vi "GFBuildMagTriggerWaveForm.vi"(3 "error in":errorcluster, 4 "Enable Array":bool[](array[boolean])=[TRUE, TRUE, TRUE, TRUE, TRUE, TRUE, TRUE], 5 "Chan Delays":dbl[](array[numeric])=[-0.8, -0.9, -0.7] format="%.6f", 6 "task in":refnum<k21>="USB-MagAndTrigFire") -> (0 "error out":errorcluster, 1 "Digital Waveform Graph":digitalwaveform[](graph), 2 "task out":refnum<k21>="USB-MagAndTrigFire")   [LabVIEW 2016]
doc: "Magnet timing pulses should be input relative to fast fire pulse, at most 2 s behind (-2 to 0 s)"
uses:
  <vilib>/Waveform/DWDTOps.llb/DWDT Boolean Array to Digital.vi
  <resource>/objmgr/daqmx.rc
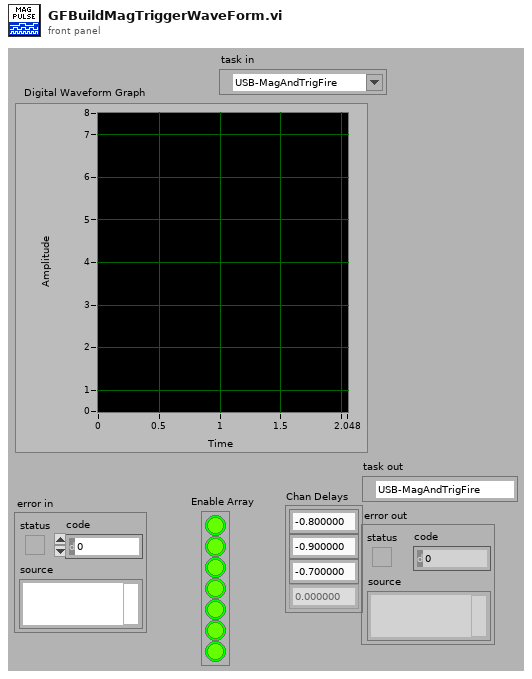
[diagram p1: front panel]
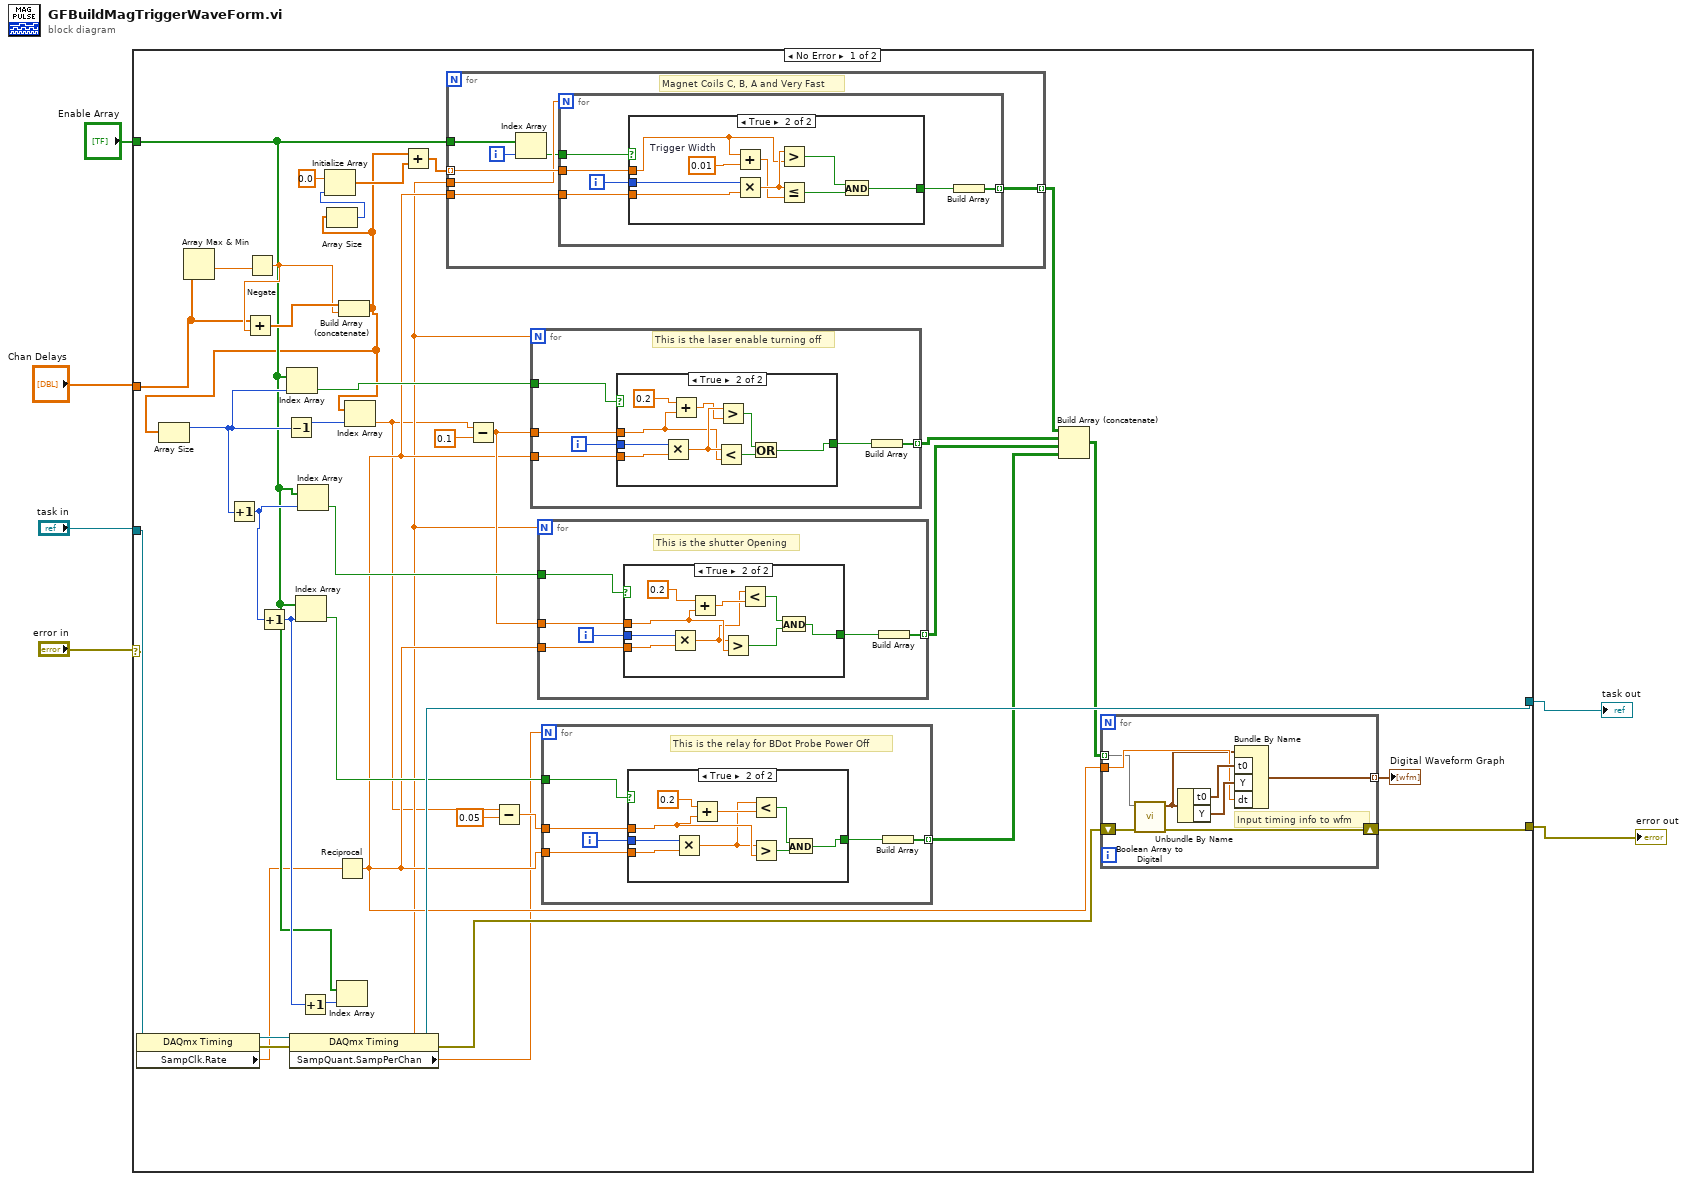
[diagram p0: block diagram]
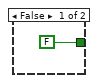
[diagram p2: hidden frame]
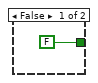
[diagram p3: hidden frame]
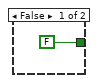
[diagram p4: hidden frame]
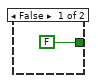
[diagram p5: hidden frame]
diagram:
  n1 = case shown="No Error" "error in" {
    selector: "error in" -> [w42 w125]
    tunnel: "task in" -> [w43 w126]
    tunnel: [w39 w126] -> w5
    tunnel: [w45 w125] -> w3
    tunnel: "Chan Delays" -> [w31 _]
    tunnel: "Enable Array" -> [w14 _]
    frame No Error {
      n2 = property class="DAQmx Timing"(reference=w43, error in=w42) -> (reference out=w41:refnum<k21>, error out=w40:errorcluster, "SampClk.Rate"=w12:dbl)
      n3 = Array Max & Min(array=w31) -> (min value=w34:dbl)  [unwired: 3 out]
      n4 = Negate(x=w34) -> (-x=w32:dbl)
      n5 = Add(x=w31, y=w32) -> (x+y=w33:dbl[])
      n6 = property class="DAQmx Timing"(reference=w41, error in=w40) -> (reference out=w39:refnum<k21>, error out=w25:errorcluster, "SampQuant.SampPerChan"=w17:dbl)
      n7 = Reciprocal(x=w12) -> (1/x=w21:dbl)
      n8 = Build Array (concatenate)(w33, w32) -> (w9:dbl[])
      n9 = Array Size(array=w9) -> (size(s)=w20:i32)
      n10 = Increment(x=w20) -> (x+1=w26:i32)
      n11 = Increment(x=w26) -> (x+1=w15:i32)
      n12 = Decrement(x=w20) -> (x-1=w38:i32)
      n13 = Index Array(array=w14, index=w20) -> (element=w30:bool)
      n14 = Index Array(array=w14, index=w15) -> (element=w24:bool)
      n15 = Index Array(array=w14, index=w26) -> (element=w28:bool)
      n16 = Increment(x=w15) -> (x+1=w16:i32)
      n17 = Array Size(array=w9) -> (size(s)=w8:i32)
      n18 = Initialize Array(0.0 ("element"), w8) -> (w10:dbl[])
      n19 = Index Array(array=w14, index=w16) -> ()  [unwired: 1 out]
      n20 = Index Array(array=w9, index=w38) -> (element=w13:dbl)
      n21 = Add(x=w9, y=w10) -> (x+y=w11:dbl[])
      n22 = for {
        tunnel: [w105] -> w36 mode=indexing
        tunnel: w11 -> [w108] mode=indexing
        tunnel: w21 -> [w107]
        tunnel: w17 -> [w106]
        tunnel: w14 -> [w104]
        i -> [w103]
        # "Magnet Coils C, B, A and Very Fast"
        n23 = Index Array(array=w104, index=w103) -> (element=w102:bool)
        n24 = for {
          N: w106 -> [_]
          tunnel: w108 -> [w113]
          tunnel: w107 -> [w114]
          tunnel: [w111] -> w105 mode=indexing
          tunnel: w102 -> [w109]
          i -> [w110]
          n25 = case shown="True" w109 {
            tunnel: w114 -> [_ w124]
            tunnel: w113 -> [_ w122]
            tunnel: [FALSE w117] -> w112
            tunnel: w110 -> [_ w116]
            frame False {
            }
            frame True {
              w121 = 0.01  # Trigger Width
              n26 = Add(x=w122, y=w121) -> (x+y=w120:dbl)
              n27 = Multiply(x=w116, y=w124) -> (x*y=w123:dbl)
              n28 = Greater?(x=w123, y=w122) -> (0:w119:bool)
              n29 = Less Or Equal?(x=w123, y=w120) -> (x <= y?=w118:bool)
              n30 = And(x=w119, y=w118) -> (x .and. y?=w117:bool)
            }
          }
          n31 = Build Array(w112) -> (w111:bool[])
        }
      }
      n32 = Subtract(x=w13, y=0.1) -> (x-y=w23:dbl)
      n33 = Subtract(x=w13, y=0.05) -> (x-y=w19:dbl)
      n34 = for {
        N: w17 -> [_]
        tunnel: w23 -> [w82]
        tunnel: w21 -> [w83]
        tunnel: [w81] -> w27 mode=indexing
        tunnel: w30 -> [w78]
        i -> [w80]
        # "This is the laser enable turning off"
        n35 = case shown="True" w78 {
          tunnel: w83 -> [_ w93]
          tunnel: w82 -> [_ w85]
          tunnel: w80 -> [_ w89]
          tunnel: [FALSE w91] -> w79
          frame False {
          }
          frame True {
            n36 = Multiply(x=w89, y=w93) -> (x*y=w88:dbl)
            n37 = Add(x=0.2, y=w85) -> (x+y=w87:dbl)
            n38 = Less?(x=w88, y=w85) -> (x < y?=w92:bool)
            n39 = Greater?(x=w88, y=w87) -> (0:w90:bool)
            n40 = Or(x=w90, y=w92) -> (x .or. y?=w91:bool)
          }
        }
        n41 = Build Array(w79) -> (w81:bool[])
      }
      n42 = for {
        N: w17 -> [_]
        tunnel: w23 -> [w66]
        tunnel: w21 -> [w67]
        tunnel: [w65] -> w29 mode=indexing
        tunnel: w28 -> [w62]
        i -> [w64]
        # "This is the shutter Opening"
        n43 = case shown="True" w62 {
          tunnel: w67 -> [_ w77]
          tunnel: w66 -> [_ w71]
          tunnel: w64 -> [_ w76]
          tunnel: [FALSE w74] -> w63
          frame False {
          }
          frame True {
            n44 = Multiply(x=w76, y=w77) -> (x*y=w69:dbl)
            n45 = Add(x=0.2, y=w71) -> (x+y=w75:dbl)
            n46 = Greater?(x=w69, y=w71) -> (0:w72:bool)
            n47 = Less?(x=w69, y=w75) -> (x < y?=w73:bool)
            n48 = And(x=w73, y=w72) -> (x .and. y?=w74:bool)
          }
        }
        n49 = Build Array(w63) -> (w65:bool[])
      }
      n50 = for {
        N: w17 -> [_]
        tunnel: w19 -> [w50]
        tunnel: w21 -> [w51]
        tunnel: [w49] -> w22 mode=indexing
        tunnel: w24 -> [w46]
        i -> [w48]
        # "This is the relay for BDot Probe Power Off"
        n51 = case shown="True" w46 {
          tunnel: w51 -> [_ w61]
          tunnel: w50 -> [_ w55]
          tunnel: w48 -> [_ w57]
          tunnel: [FALSE w59] -> w47
          frame False {
          }
          frame True {
            n52 = Multiply(x=w57, y=w61) -> (x*y=w53:dbl)
            n53 = Add(x=0.2, y=w55) -> (x+y=w54:dbl)
            n54 = Less?(x=w53, y=w54) -> (x < y?=w58:bool)
            n55 = Greater?(x=w53, y=w55) -> (0:w60:bool)
            n56 = And(x=w58, y=w60) -> (x .and. y?=w59:bool)
          }
        }
        n57 = Build Array(w47) -> (w49:bool[])
      }
      n58 = Build Array (concatenate)(w36, w27, w29, w22) -> (w35:bool[][][])
      n59 = for {
        shift-right: [w101] -> w45
        shift-left: w25 -> [w100]
        tunnel: w35 -> [w94] mode=indexing
        tunnel: [w95] -> w44 mode=indexing
        tunnel: w21 -> [w97]
        # "Input timing info to wfm"
        n60 = call-poly <vilib>:"Boolean Array to Digital.vi"("error in (no error)"=w100, "boolean array"=w94) -> ("error out"=w101:errorcluster, "digital waveform"=w96:digitalwaveform)  [unwired: 8 in]
        n61 = Unbundle By Name(w96) -> ("t0"=w99:timestamp, "Y"=w98:digitaldata)
        n62 = Bundle By Name(cluster=w96, "t0"=w99, "Y"=w98, "dt"=w97) -> (w95:digitalwaveform)
      }
      "Digital Waveform Graph" <- w44
    }
    frame Error {
    }
  }
  "error out" <- w3
  "task out" <- w5
